vi "Modulation Measurement.vi"() -> ()   [LabVIEW 2013]
uses:
  <vilib>/Utility/file.llb/Write To Spreadsheet File (DBL).vi
  <instrlib>/Agilent 33XXX Series/Agilent 33XXX Series.lvlib
  <instrlib>/Tektronix TDS 200 1000 2000 Series/Tektronix TDS 200 1000 2000 Series.lvlib
panel:
  out "Waveform Graph":dbl[](graph)
  in  "Stop":dbl format="%#_13g"
  in  "Stepsize":dbl format="%#_13g"
  in  "Start":dbl format="%#_13g"
  out "Measurement":dbl
  in  "Enable Output  (T: Enable)":bool=TRUE
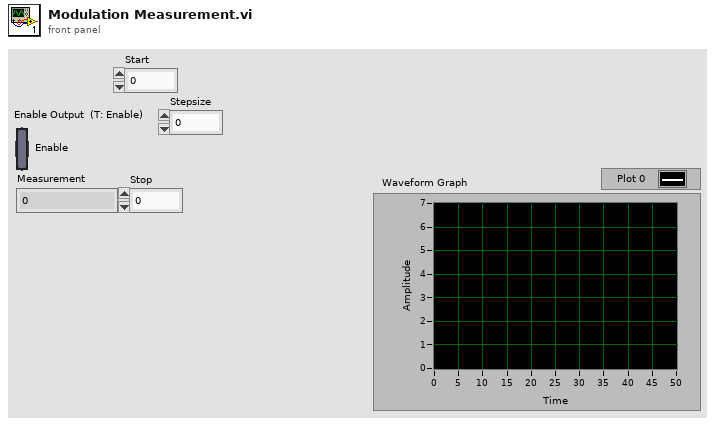
[diagram p1: front panel]
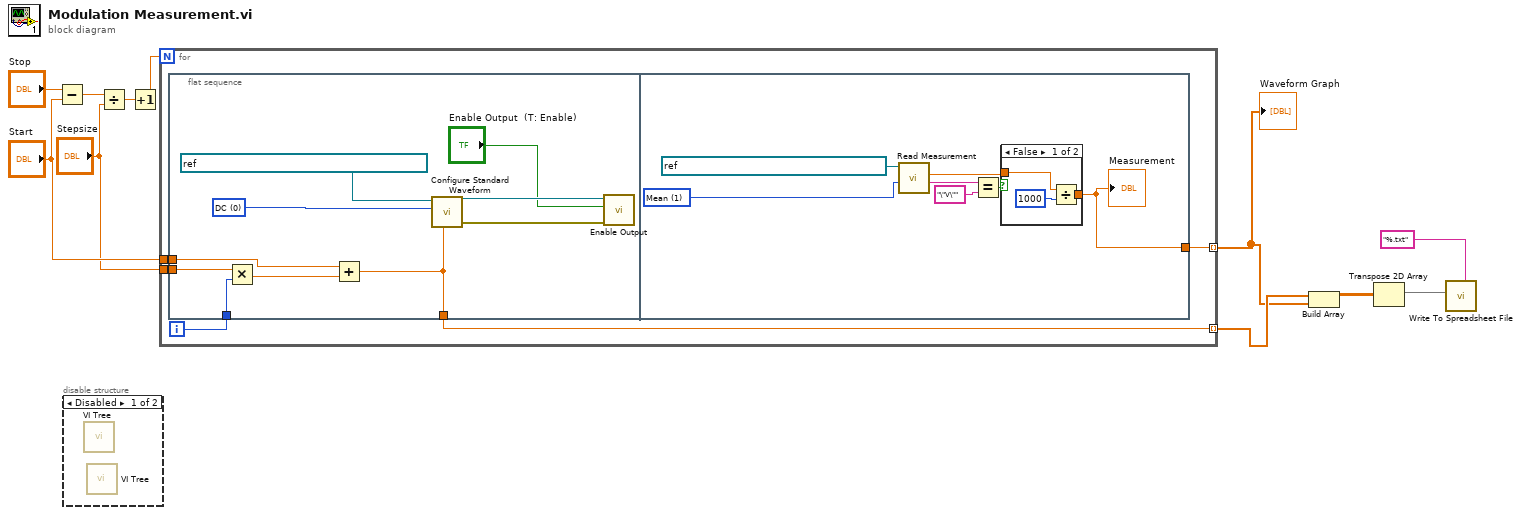
[diagram p0: block diagram]
diagram:
  n1 = Subtract(x="Stop", y="Start") -> (x-y=w9:dbl)
  n2 = disable-structure shown="Disabled" {
    frame Disabled {
      n3 = call <instrlib>:"VI Tree.vi"() -> ()  [unwired: 12 in]
      n4 = call <instrlib>:"VI Tree.vi"() -> ()  [unwired: 12 in]
    }
    frame Enabled {
    }
  }
  n5 = Divide(x=w9, y="Stepsize") -> (x/y=w7:dbl)
  n6 = Increment(x=w7) -> (x+1=w6:dbl)
  n7 = for {
    N: w6 -> [_]
    tunnel: "Start" -> [w16]
    tunnel: "Stepsize" -> [w15]
    tunnel: [w13] -> w4 mode=indexing
    tunnel: [w12] -> w5 mode=indexing
    i -> [w14]
    n8 = flat-sequence {
      tunnel: w16 -> [w21]
      tunnel: w15 -> [w19]
      tunnel: w14 -> [w18]
      tunnel: [w17] -> w12
      tunnel: [w27] -> w13
      frame #0 {
        w26 = u16 0 items=["DC", "Sine", "Square", "Triangle", "Ramp", "Pulse", "Noise", "Sinc", "Negative Ramp", "Exponential Rise", "Exponential Fall", "Cardiac"] ("Waveform Function (1: Sine)")
        n9 = Multiply(x=w19, y=w18) -> (x*y=w20:dbl)
        n10 = Add(x=w21, y=w20) -> (x+y=w17:dbl)
        n11 = call <instrlib>:"Configure Standard Waveform.vi"("DC Offset (0.00 V)"=w17, "Waveform Function (1: Sine)"=w26, "VISA resource name"=refnum<visa-resource-name> "USB0::0x0957::0x1507::MY48004204::INSTR") -> ("error out"=w23:errorcluster, "VISA resource name out"=w24:refnum<visa-resource-name>)  [unwired: 7 in]
        n12 = call <instrlib>:"Enable Output.vi"("error in (no error)"=w23, "Enable Output  (T: Enable)"="Enable Output  (T: Enable)", "VISA resource name"=w24) -> ()  [unwired: 7 in, 2 out]
      }
      frame #1 {
        w28 = 1 items=["Frequency", "Mean", "Period", "Pulse Duty", "Peak to Peak", "Cycle RMS", "Minimum", "Maximum", "Rise Time", "Fall Time", "Positive Width", "Negative Width", "Amplitude", "Cycle Mean", "High", "Low", "Negative Duty", "Positive Overshoot", "Negative Overshoot", "Cursor Mean", "Burst Width", "Positive Pulse Count", "Negative Pulse Count", "Rising Edge Count", "Falling Edge Count", "Area", "Cycle Area", "RMS", "Cursor RMS"] ("Measurement Type (0: Frequency)")
        n13 = call <instrlib>:"Read Measurement.vi"("Measurement Type (0: Frequency)"=w28, "VISA resource name"=refnum<visa-resource-name> "USB0::0x0699::0x0362::C102704::INSTR") -> ("Units"=w31:string, "Measurement"=w33:dbl)  [unwired: 6 in, 2 out]
        n14 = Equal?(x=w31, y="\"V\"") -> (x = y?=w32:bool)
        n15 = case shown="False" w32 {
          tunnel: w33 -> [w35 w37]
          tunnel: [w34 w37] -> w27
          frame False {
            n16 = Divide(x=w35, y=1000) -> (x/y=w34:dbl)
          }
          frame True {
          }
        }
        "Measurement" <- w27
      }
    }
  }
  "Waveform Graph" <- w4
  n17 = Build Array(w5, w4) -> (w3:dbl[][])
  n18 = Transpose 2D Array(2D array=w3) -> (transposed array=w2:dbl[][])
  n19 = call-poly <vilib>:"Write To Spreadsheet File.vi"("format (%.3f)"="%.txt", "2D data"=w2) -> ()  [unwired: 6 in, 1 out]
